vi "Plot Closed.vi"(8 "error in (no error)":errorcluster, 10 "Closed plot":refnum<class "Message Enqueuer.lvclass">, 11 "Monitor-Pulse in":refnum<class "Monitor-Pulse.lvclass">) -> (0 "error out":errorcluster, 3 "Monitor-Pulse out":refnum<class "Monitor-Pulse.lvclass">)   [LabVIEW 2016, in "Monitor-Pulse.lvclass"]
uses:
  Monitor-Pulse.lvclass
  <vilib>/ActorFramework/Message Enqueuer/Message Enqueuer.lvclass
  Monitor-Pulse.lvclass/Monitor-Pulse.ctl
  Measure_core/Controllers/Process Controller/Process Controller.lvclass
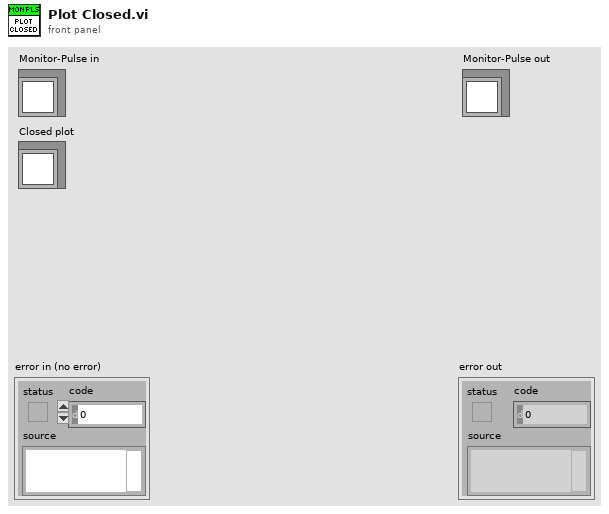
[diagram p1: front panel]
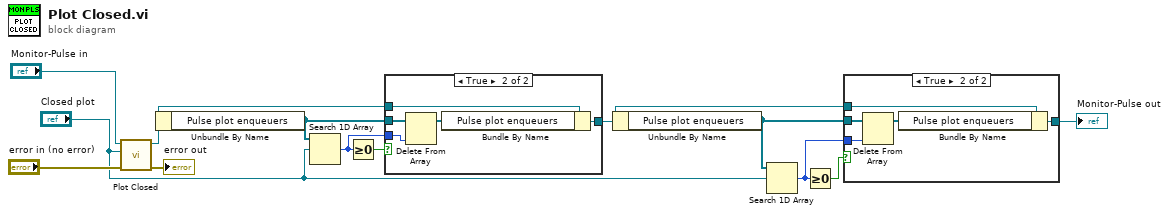
[diagram p0: block diagram]
diagram:
  n1 = call-parent "Plot Closed.vi"("error in (no error)"="error in (no error)", "Closed plot"="Closed plot", "Measure Controller in"="Monitor-Pulse in") -> ("error out"=→"error out":errorcluster, "Measure Controller out"=w7:refnum<class "Monitor-Pulse.lvclass">)  [unwired: 7 in]
  n2 = Unbundle By Name(w7) -> ("Pulse plot enqueuers"=w10:refnum<class "Message Enqueuer.lvclass">[])
  n3 = Search 1D Array(1D array=w10, element="Closed plot") -> (index of element=w9:i32)  [unwired: 1 in]
  n4 = Greater Or Equal To 0?(x=w9) -> (x >= 0?=w8:bool)
  n5 = case shown="True" w8 {
    tunnel: w10 -> [_ w19]
    tunnel: w9 -> [_ w18]
    tunnel: w7 -> [w14 w17]
    tunnel: [w14 w15] -> w2
    frame False {
    }
    frame True {
      n6 = Delete From Array(array=w19, index=w18) -> (array with subset deleted=w16:refnum<class "Message Enqueuer.lvclass">[])  [unwired: 1 in, 1 out]
      n7 = Bundle By Name(cluster=w17, "Pulse plot enqueuers"=w16) -> (w15:refnum<class "Monitor-Pulse.lvclass">)
    }
  }
  n8 = Unbundle By Name(w2) -> ("Pulse plot enqueuers"=w6:refnum<class "Message Enqueuer.lvclass">[])
  n9 = Search 1D Array(1D array=w6, element="Closed plot") -> (index of element=w5:i32)  [unwired: 1 in]
  n10 = Greater Or Equal To 0?(x=w5) -> (x >= 0?=w4:bool)
  n11 = case shown="True" w4 {
    tunnel: w6 -> [_ w25]
    tunnel: w5 -> [_ w24]
    tunnel: w2 -> [w20 w23]
    tunnel: [w20 w21] -> w1
    frame False {
    }
    frame True {
      n12 = Delete From Array(array=w25, index=w24) -> (array with subset deleted=w22:refnum<class "Message Enqueuer.lvclass">[])  [unwired: 1 in, 1 out]
      n13 = Bundle By Name(cluster=w23, "Pulse plot enqueuers"=w22) -> (w21:refnum<class "Monitor-Pulse.lvclass">)
    }
  }
  "Monitor-Pulse out" <- w1
